vi "DSF.Engine.Execution.Transfer.RT FIFO.Data.From.vi"(8 "error in (no error)":errorcluster, 10 "Transfer Data":T1 {"Buffer Descriptor"."address" format="%016x"; "Buffer Descriptor"."size" format="%d bytes"}, 11 "Transfer in":refnum<class "DSF.Engine.Execution.Transfer.lvclass">) -> (0 "error out":errorcluster, 3 "Transfer out":refnum<class "DSF.Engine.Execution.Transfer.lvclass">)   [LabVIEW 2016, in "DSF.Engine.lvlib" / "DSF.Engine.Execution.Transfer.lvclass"]
uses:
  DSF.Engine.Execution.Transfer.lvclass
  DSF.Engine.Execution.Transfer.RT FIFO Data.ctl
  DSF.Engine.Execution.Transfer.lvclass/DSF.Engine.Execution.Transfer.ctl
  Buffer/DSF.Engine.Memory.Buffer.lvclass
  C:/Git/SourceTree/DSF/Source/Submodules/Memory/Source/Classes/Pointer/Memory.Pointer.lvclass
  Submodules/Memory/Source/Classes/Pointer/Memory.Pointer.lvclass/Memory.Pointer.ctl
  Submodules/Memory/Source/Classes/Pointer/Memory.Pointer.Block Descriptor to Object.vi
  Submodules/Memory/Source/Classes/Pointer/Memory.Pointer.Set Address.vi
  Submodules/Memory/Source/Classes/Pointer/Memory.Pointer.Set Size.vi
  Submodules/Memory/Source/Classes/Pointer/Memory.Pointer.Parameter Check.Null Pointer.vi
  Submodules/Memory/Source/Classes/Pointer/Memory.Pointer.Errors.vi
  Submodules/Memory/Source/Classes/Pointer/Memory.Pointer.Errors.Null Pointer.vi
  Submodules/Memory/Source/Classes/Pointer/Memory.Pointer.Get Address.vi
  Submodules/Memory/Source/Classes/Pointer/Memory.Pointer.Errors.Create Error.vi
  Submodules/Memory/Source/Submodules/SEH/Source/VIs/Static Error Handling.Error Cluster Constant.vi
  Submodules/Memory/Source/Submodules/SEH/Source/VIs/Static Error Handling.Error Cluster Constant (256B).vi
  Submodules/Memory/Source/Submodules/SEH/Source/VIs/Static Error Handling.Parameters.Status.Set.vi
  Submodules/Memory/Source/Submodules/SEH/Source/VIs/Static Error Handling.Parameters.Code.Set.vi
  Submodules/Memory/Source/Submodules/SEH/Source/VIs/Static Error Handling.Parameters.VI Source.Set.vi
  Submodules/Memory/Source/Constants/Memory.Constants.vi
  Submodules/Memory/Source/Constants/Memory.Constants.Library Name.vi
  Submodules/Memory/Source/Classes/Pointer/Memory.Pointer.Errors.Get Info.vi
  Submodules/Memory/Source/Submodules/SEH/Source/VIs/Static Error Handling.Source Buffer.Write.String.vi
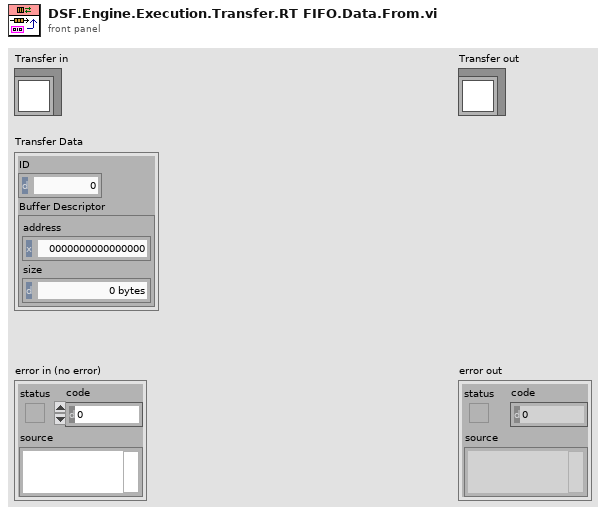
[diagram p1: front panel]
types:
  T1 = typedef "DSF.Engine.lvlib/DSF.Engine.Execution.Transfer.lvclass/DSF.Engine.Execution.Transfer.RT FIFO Data.ctl" = cluster{"ID":i32, "Buffer Descriptor":cluster{"address":u64, "size":u64}}
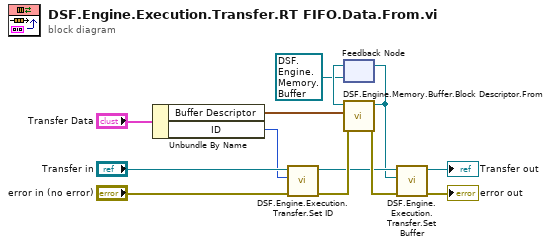
[diagram p0: block diagram]
diagram:
  n1 = Unbundle By Name("Transfer Data") -> ("Buffer Descriptor"=w9:cluster{"address":u64, "size":u64}, "ID"=w10:i32)
  n2 = call "DSF.Engine.Execution.Transfer.Set ID.vi"("error in (no error)"="error in (no error)", "id"=w10, "Transfer in"="Transfer in") -> ("error out"=w8:errorcluster, "Transfer out"=w2:refnum<class "DSF.Engine.Execution.Transfer.lvclass">)  [unwired: 7 in]
  n3 = feedback #1(refnum<class "DSF.Engine.Memory.Buffer.lvclass"> refnum ("Buffer out")) -> (w7:refnum<class "DSF.Engine.Memory.Buffer.lvclass">)
  n4 = call "DSF.Engine.Memory.Buffer.Block Descriptor.From.vi"("error in (no error)"=w8, "block descriptor"=w9, "Buffer in"=w7) -> ("error out"=w3:errorcluster, "Buffer out"=w1:refnum<class "DSF.Engine.Memory.Buffer.lvclass">)  [unwired: 7 in]
  n5 = feedback-in #1(w1) -> ()
  n6 = call "DSF.Engine.Execution.Transfer.Set Buffer.vi"("error in (no error)"=w3, "Buffer"=w1, "Transfer in"=w2) -> ("error out"=→"error out":errorcluster, "Transfer out"=→"Transfer out":refnum<class "DSF.Engine.Execution.Transfer.lvclass">)  [unwired: 7 in]
